vi "Statistics Parameters_SM.vi"(8 "error in (no error)":errorcluster, 10 "StatisticalParameters":string[][](array[string]), 11 "Inspection Statemachine in":refnum<class "Inspection Statemachine.lvclass">) -> (0 "error out":errorcluster, 3 "Inspection Statemachine out":refnum<class "Inspection Statemachine.lvclass">)   [LabVIEW 2019, in "Inspection Statemachine.lvclass"]
uses:
  Inspection Statemachine.lvclass
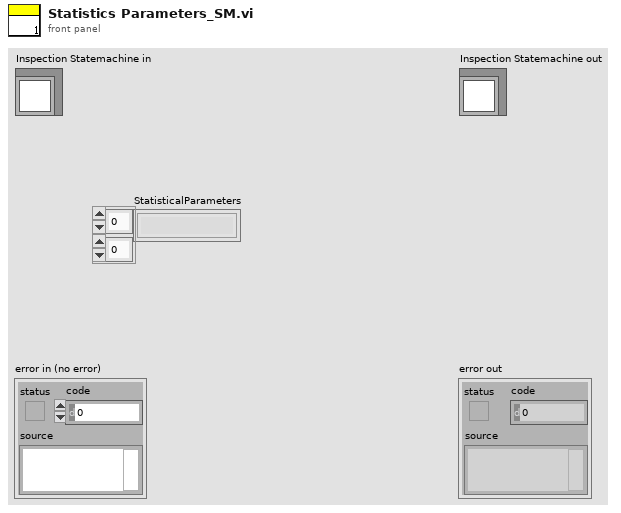
[diagram p1: front panel]
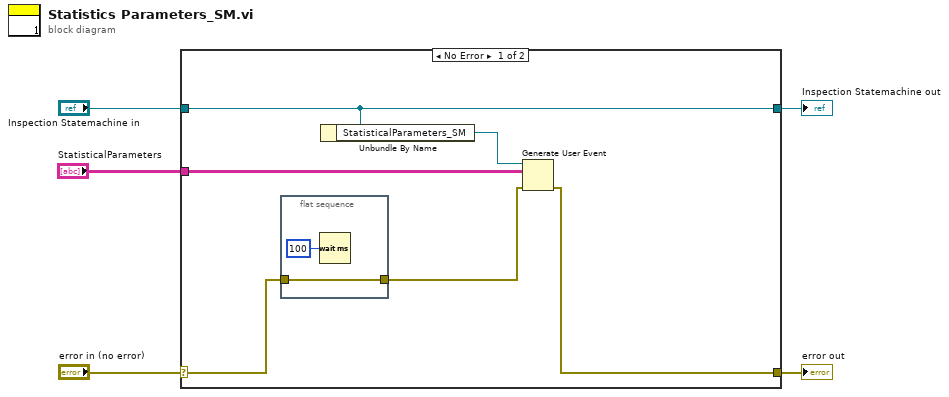
[diagram p0: block diagram]
diagram:
  n1 = case shown="No Error" "error in (no error)" {
    selector: "error in (no error)" -> [w7 w15]
    tunnel: [w8 w15] -> w4
    tunnel: [w11 w14] -> w2
    tunnel: "Inspection Statemachine in" -> [w11 w14]
    tunnel: "StatisticalParameters" -> [w9 _]
    frame No Error {
      n2 = flat-sequence {
        tunnel: [w13] -> w6
        tunnel: w7 -> [w13]
        frame #0 {
          n3 = Wait (ms)(milliseconds to wait=u32 100) -> ()  [unwired: 1 out]
        }
      }
      n4 = Unbundle By Name(w11) -> ("StatisticalParameters_SM"=w10:refnum<user-event>)
      n5 = Generate User Event(user event=w10, event data cluster=w9, error in=w6) -> (error out=w8:errorcluster)  [unwired: 1 in, 1 out]
    }
    frame Error {
    }
  }
  "error out" <- w4
  "Inspection Statemachine out" <- w2
